vi "Acquire.vi"(8 "error in (no error)":errorcluster, 10 "Msg in":T1, 11 "PXIDigitizer in":refnum<class "Ztec4611.lvclass">) -> (0 "error out":errorcluster, 1 "new command":string, 2 "Msg out":T1, 3 "PXIDigitizer out":refnum<class "Ztec4611.lvclass">)   [LabVIEW 2011, in "Ztec4611.lvclass"]
uses:
  Ztec4611.lvclass
  DriverMsg.ctl
  Ztec4611.lvclass/Ztec4611.ctl
  BaseDriver/BaseDriver.lvclass
  PXIDigitizer.lvclass
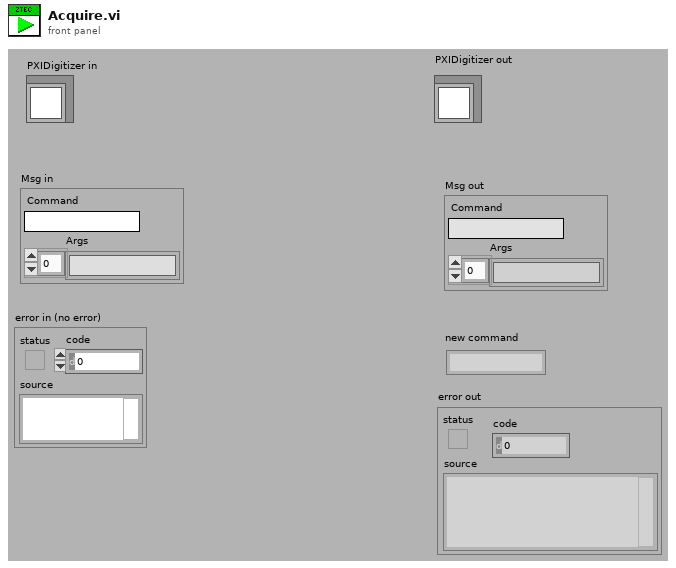
[diagram p1: front panel]
types:
  T1 = typedef "DriverMsg.ctl" = cluster{"Command":string, "Args":string[]}
  T2 = typedef "OnOffTypeDef.ctl" = enum16{"off", "on"}
  T3 = cluster{"actualSamples":i32, "absoluteInitialX":dbl, "relativeInitialX":dbl, "xIncrement":dbl, "offset":dbl, "gain":dbl, "reserved1":dbl, "reserved2":dbl}[]
  T4 = typedef "MeasurementsCluster_TypDEf.ctl" = cluster{"Analysis1":dbl, "Analysis2":dbl, "Analysis3":dbl, "Analysis4":dbl, "Analysis5":dbl, "Analysis6":dbl, "Analysis7":dbl, "Analysis8":dbl, "Analysis9":dbl, "Analysis10":dbl}
  T5 = typedef "methodCluster_TypDEf.ctl" = cluster{"Analysis1":T6, "Analysis2":T6, "Analysis3":T6, "Analysis4":T6, "Analysis5":T6, "Analysis6":T6, "Analysis7":T6, "Analysis8":T6, "Analysis9":T6, "Analysis10":T6}
  T6 = typedef "method_TypDef.ctl" = enum16{"n/a", "max", "min", "energy"}
  T7 = typedef "LinkedChannelsCluster_TypDef.ctl" = cluster{"Analysis1":T8, "Analysis2":T8, "Analysis3":T8, "Analysis4":T8, "Analysis5":T8, "Analysis6":T8, "Analysis7":T8, "Analysis8":T8, "Analysis9":T8, "Analysis10":T8}
  T8 = typedef "channels_TypDef.ctl" = enum16{"Channel0", "Channel1", "Channel2", "Channel3", "Channel4", "Channel5", "Channel6", "Channel7", "n/a"}
  T9 = cluster{"Channel0":string, "Channel1":string, "Channel2":string, "Channel3":string, "Channel4":string, "Channel5":string, "Channel6":string, "Channel7":string}
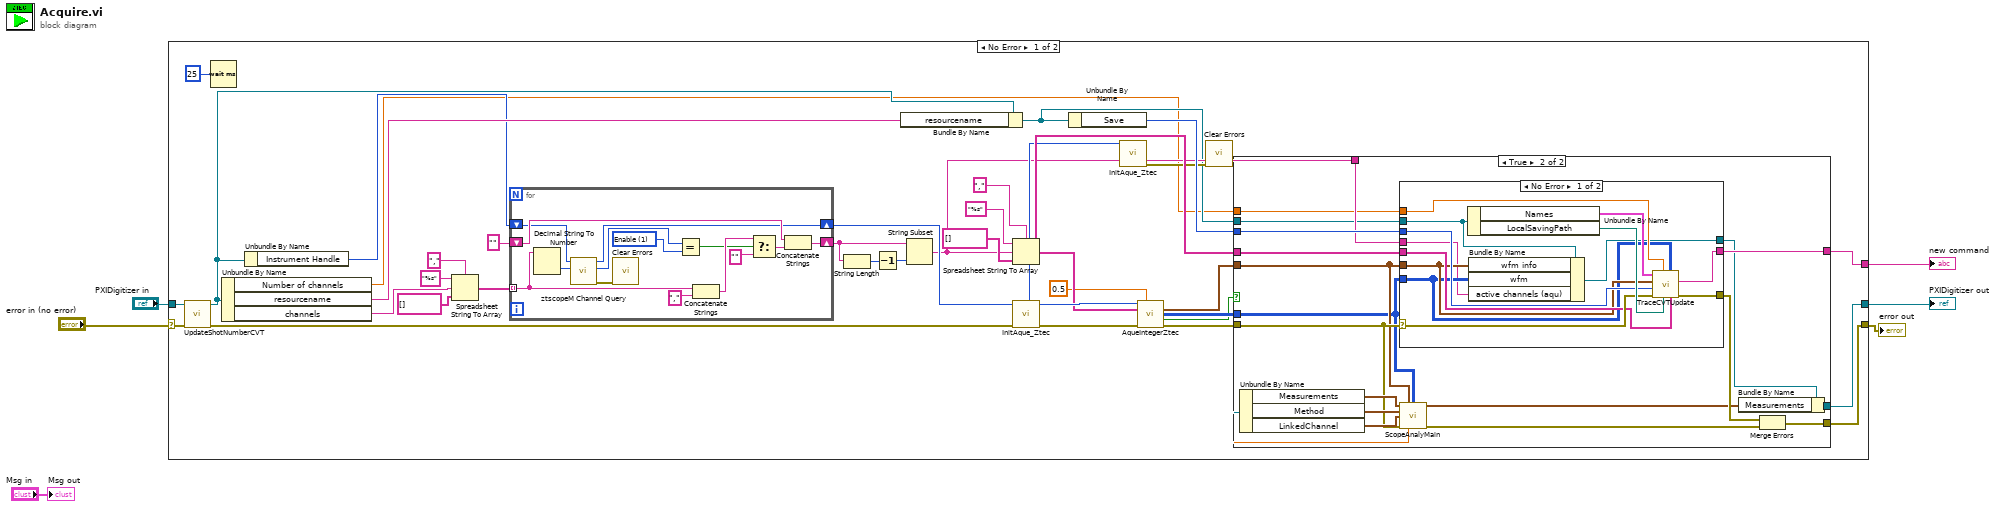
[diagram p0: block diagram]
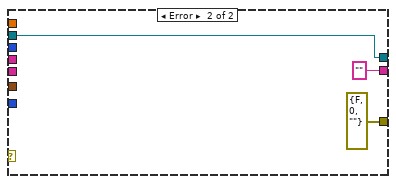
[diagram p3: hidden frame]
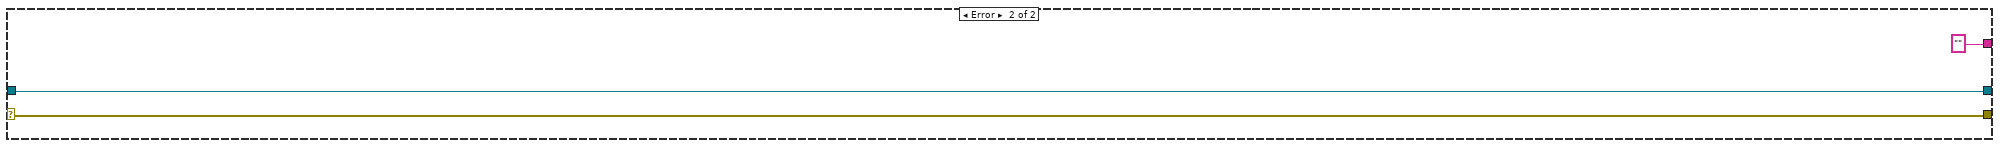
[diagram p4: hidden frame]
diagram:
  n1 = case shown="No Error" "error in (no error)" {
    selector: "error in (no error)" -> [w36 w95]
    tunnel: "PXIDigitizer in" -> [w43 w96]
    tunnel: [w9 w96] -> w6
    tunnel: [w12 w95] -> w4
    tunnel: [w24 "" ("new command")] -> w1
    frame No Error {
      n2 = call "UpdateShotNumberCVT.vi"("error in (no error)"=w36, "BaseDriver in"=w43) -> ("error out"=w22:errorcluster, "BaseDriver out"=w37:refnum<class "Ztec4611.lvclass">)  [unwired: 8 in]
      n3 = Wait (ms)(milliseconds to wait=u32 25) -> ()  [unwired: 1 out]
      n4 = Unbundle By Name ("pressure read")(w37) -> ("Number of channels"=w10:dbl, "resourcename"=w42:string, "channels"=w40:string)
      n5 = Unbundle By Name(w37) -> ("Instrument Handle"=w34:i32)
      n6 = Spreadsheet String To Array(delimiter (Tab)=",", format string="%s", spreadsheet string=w40, array type (2D Dbl)=string[] []) -> (array=w30:string[])
      n7 = for {
        shift-right: [w86] -> w23
        shift-left: w34 -> [w87]
        tunnel: w30 -> [w82] mode=indexing
        shift-right: [w89] -> w26
        shift-left: "" -> [w88]
        w85 = 1 items=["Enable"=1, "Disable"=0] ("State")
        n8 = Decimal String To Number(string=w82) -> (number=w81:i32)  [unwired: 2 in, 1 out]
        n9 = call "ztscopeM Channel Query.vi"("Channel"=w81, "Instrument Handle In"=w87) -> ("error out"=w80:errorcluster, "State"=w84:i32, "Instrument Handle Out"=w86:i32)  [unwired: 7 in]
        n10 = call "Clear Errors.vi"("error in (no error)"=w80) -> ()  [unwired: 6 in, 1 out]
        n11 = Equal?(x=w84, y=w85) -> (x = y?=w83:bool)
        n12 = Concatenate Strings(w82, "," ("string")) -> (w91:string)
        n13 = Select(t=w91, s=w83, f="") -> (s? t:f=w90:string)
        n14 = Concatenate Strings(w88, w90) -> (w89:string)
      }
      n15 = String Length(string=w26) -> (length=w28:i32)
      n16 = Decrement(x=w28) -> (x-1=w27:i32)
      n17 = Bundle By Name(cluster=w37, "resourcename"=w42) -> (w14:refnum<class "Ztec4611.lvclass">)
      n18 = String Subset(string=w26, length (rest)=w27) -> (substring=w15:string)  [unwired: 1 in]
      n19 = Spreadsheet String To Array(delimiter (Tab)=",", format string="%s", spreadsheet string=w15, array type (2D Dbl)=string[] []) -> (array=w20:string[])
      n20 = call "InitAque_Ztec.vi"("error in (no error)"=w22, "Instrument Handle Out in"=w23) -> ("error out"=w18:errorcluster, "Instrument Handle Out out"=w21:i32)  [unwired: 8 in]
      n21 = Unbundle By Name(w14) -> ("Save"=w25:T2)
      n22 = call "AqueIntegerZtec.vi"("Instrument Handle in"=w21, "timeout (s)"=0.5 ("timeout"), "Active Channel Array"=w20, "error in (no error)"=w18) -> ("Instrument Handle Out"=w16:i32, "wfm info"=w11:T3, "wfm"=w8:i16[][], "Aque OK"=w7:bool, "error out"=w13:errorcluster)  [unwired: 7 in]
      n23 = call "InitAque_Ztec.vi"("Instrument Handle Out in"=w16) -> ("error out"=w17:errorcluster)  [unwired: 9 in, 1 out]
      n24 = call "Clear Errors.vi"("error in (no error)"=w17) -> ()  [unwired: 6 in, 1 out]
      n25 = case shown="True" w7 {
        tunnel: w25 -> [_ w63]
        tunnel: [_ w62] -> w24
        tunnel: w20 -> [_ w61]
        tunnel: w15 -> [_ w60]
        tunnel: w14 -> [w45 w59]
        tunnel: w13 -> [w44 w55]
        tunnel: [w44 w52] -> w12
        tunnel: w11 -> [_ w51]
        tunnel: w10 -> [_ w50]
        tunnel: [w45 w47] -> w9
        tunnel: w8 -> [_ w46]
        frame False {
        }
        frame True {
          n26 = Unbundle By Name ("pressure read")(w59) -> ("Measurements"=w58:T4, "Method"=w57:T5, "LinkedChannel"=w56:T7)
          n27 = case shown="No Error" w55 {
            selector: w55 -> [w74 _]
            tunnel: w51 -> [w68 _]
            tunnel: w46 -> [w67 _]
            tunnel: w61 -> [w71 _]
            tunnel: w63 -> [w73 _]
            tunnel: w59 -> [w69 w77]
            tunnel: [w70 "" ("String")] -> w62
            tunnel: [w65 errorcluster {"status"=FALSE, "code"=0, "source"=""} ("error IO")] -> w54
            tunnel: [w66 w77] -> w49
            tunnel: w50 -> [w72 _]
            tunnel: w60 -> [w64 _]
            frame No Error {
              n28 = Unbundle By Name ("pressure read")(w69) -> ("Names"=w76:T9, "LocalSavingPath"=w75:path)
              n29 = Bundle By Name(cluster=w69, "wfm info"=w68, "wfm"=w67, "active channels (aqu)"=w64) -> (w66:refnum<class "Ztec4611.lvclass">)
              n30 = call "TraceCVTUpdate.vi"("Array"=w71, "wfm"=w67, "Settings.LocalSavingPath"=w75, "Number of channels"=w72, "error in (no error)"=w74, "Save"=w73, "wfm info"=w68, "Settings.Names"=w76) -> ("error out"=w65:errorcluster, "String out"=w70:string)  [unwired: 1 in, 1 out]
            }
            frame Error {
            }
          }
          n31 = call "ScopeAnalyMain.vi"("Measurements"=w58, "wfm info"=w51, "wfm"=w46, "Method"=w57, "LinkedChannel"=w56, "error in (no error)"=w55, "Number of channels"=w50) -> ("Measurements"=w48:T4, "error out"=w53:errorcluster)  [unwired: 7 in]
          n32 = Bundle By Name(cluster=w49, "Measurements"=w48) -> (w47:refnum<class "Ztec4611.lvclass">)
          n33 = Merge Errors(w54, w53) -> (w52:errorcluster)
        }
      }
    }
    frame Error {
    }
  }
  "PXIDigitizer out" <- w6
  "error out" <- w4
  "new command" <- w1
  "Msg out" <- "Msg in"
